vi "Get Available Components 1.0.vi"(8 "error in (no error)":errorcluster, 10 "Include Hidden (F)":bool, 11 "Session in":refnum<k21>) -> (0 "error out":errorcluster, 2 "Software Components":T1[](array[typedef]), 3 "Session out":refnum<k21>)   [LabVIEW 2020, in "nisyscfg.lvlib"]
uses:
  <vilib>/nisyscfg/nisyscfg.lvlib
  <vilib>/nisyscfg/Software.ctl
  <vilib>/nisyscfg/Component Types.ctl
  <vilib>/nisyscfg/Get Available Components.vi
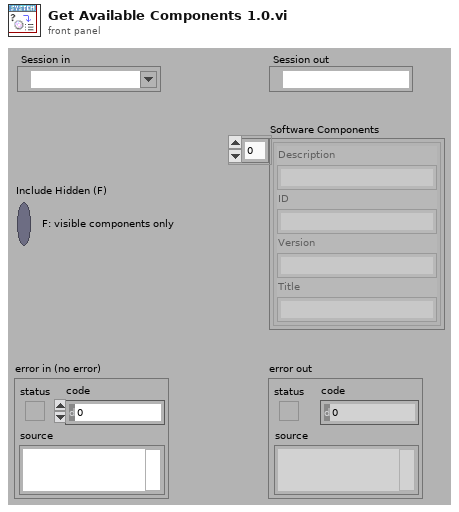
[diagram p1: front panel]
types:
  T1 = typedef "nisyscfg.lvlib/Software.ctl" = cluster{"Description":string, "ID":string, "Version":string, "Title":string}
  T2 = typedef "nisyscfg.lvlib/Component Types.ctl" = u32
  T3 = typedef "nisyscfg.lvlib/Software 1.2.ctl" = cluster{"title":string, "description":string, "ID":string, "version":string, "component type":T4}
  T4 = typedef "nisyscfg.lvlib/Component Type.ctl" = u32
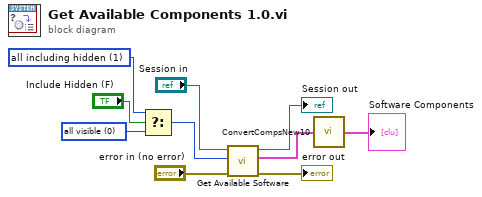
[diagram p0: block diagram]
diagram:
  w5 = T2 0 items=["all visible", "all including hidden"] ("component types")
  w6 = T2 1 items=["all visible", "all including hidden"] ("component types")
  n1 = Select(t=w6, s="Include Hidden (F)", f=w5) -> (s? t:f=w3:T2)
  n2 = call-poly <vilib>:"Get Available Software.vi"("error in (no error)"="error in (no error)", "Item Types (all visible)"=w3, "Session in"="Session in") -> ("error out"=→"error out":errorcluster, "Software Components"=w1:T3[], "Session out"=→"Session out":refnum<k21>)  [unwired: 6 in]
  n3 = call <vilib>:"ConvertCompsNew10.vi"("components 1.2"=w1) -> ("components 1.0"=→"Software Components":T1[])
